vi "StringifiedData.vi"(8 "error in (no error)":errorcluster, 11 "StringMsg in":refnum<class "StringMsg.lvclass">) -> (0 "error out":errorcluster, 2 "Stringified Data":string, 3 "StringMsg out":refnum<class "StringMsg.lvclass">)   [LabVIEW 2017, in "LapDog.Messaging.v3.NativeTypes.lvlib" / "StringMsg.lvclass"]
doc: "This VI is used for the message probe. Child classes may override it and provide the message data in string format or a short string describing the data the message contains. This string will be displayed in the probe window."
uses:
  StringMsg.lvclass
  StringMsg.lvclass/StringMsg.ctl
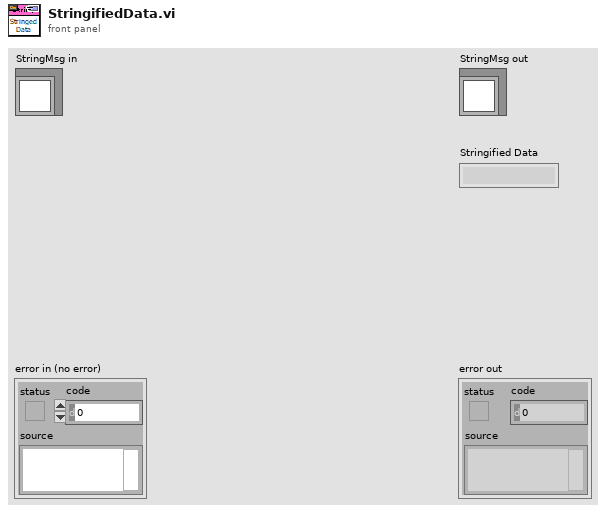
[diagram p1: front panel]
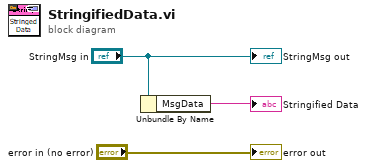
[diagram p0: block diagram]
diagram:
  n1 = Unbundle By Name("StringMsg in") -> ("MsgData"=→"Stringified Data":string)
  "error out" <- "error in (no error)"
  "StringMsg out" <- "StringMsg in"
